vi "alg_multiplication (SubVI).vi"(8 "에러 입력(에러 없음)":errorcluster, 10 "b":dbl[][](array[numeric])=[[1.0, 1.0], [1.0, 1.0]], 11 "a":dbl[][](array[numeric])=[[1.0, 1.0]]) -> (0 "에러 출력":errorcluster, 2 "ans":dbl[][](array[numeric]), 3 "참조 번호 출력":refnum<k35>)   [LabVIEW 2018]
uses:
  PythonConfigGlobal.vi
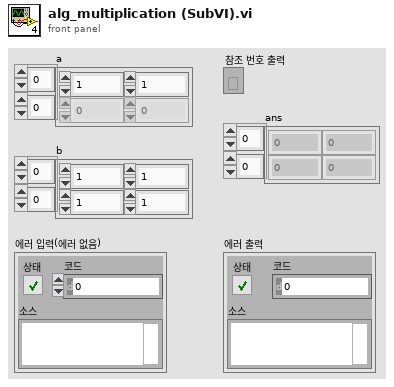
[diagram p1: front panel]
types:
  T1 = cluster{"session out":refnum<k35>, "appended path":path}
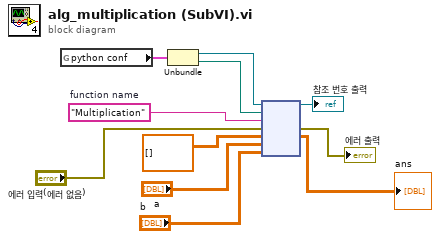
[diagram p0: block diagram]
diagram:
  w1 = "Multiplication"  # function name
  n1 = global read "PythonConfigGlobal.vi" "python conf"() -> (w8:T1)
  n2 = Unbundle(w8) -> ("session out"=w6:refnum<k35>, "appended path"=w7:path)
  n3 = node(w6, w7, w1, "에러 입력(에러 없음)", dbl[][] [] ("str1"), "a", "b") -> (→"참조 번호 출력":refnum<k35>, →"에러 출력":errorcluster, →"ans":dbl[][])  [unwired: 2 in, 2 out]
